vi "Get Base Protocol.vi"(8 "error in (no error)":errorcluster, 11 "UDP in":refnum<class "UDP.lvclass">) -> (0 "error out":errorcluster, 2 "Protocol out":T1, 3 "UDP out":refnum<class "UDP.lvclass">)   [LabVIEW 2019, in "Protocols.lvlib" / "UDP.lvclass"]
uses:
  UDP.lvclass
  Protocol Parent/Types/Base Protocol Type.ctl
  Protocol Parent/Protocol Parent.lvclass
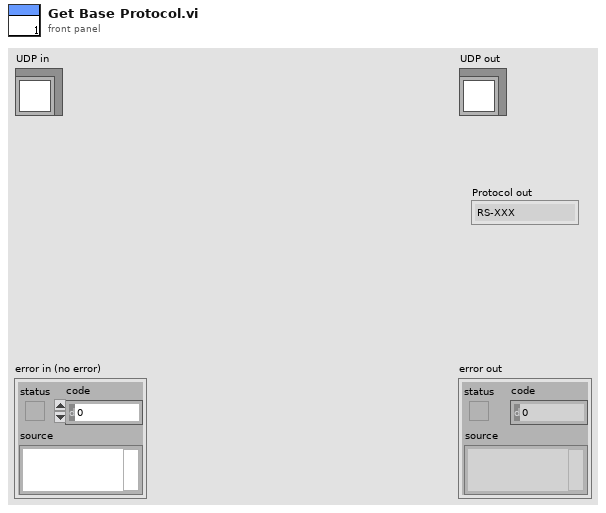
[diagram p1: front panel]
types:
  T1 = typedef "Protocols.lvlib/Protocol Parent.lvclass/Base Protocol Type.ctl" = enum16{"RS-XXX", "VISA", "TCPIP", "UDP"}
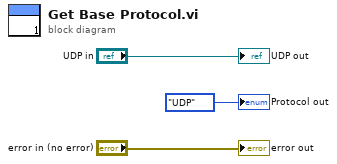
[diagram p0: block diagram]
diagram:
  "error out" <- "error in (no error)"
  "UDP out" <- "UDP in"
  "Protocol out" <- Base_Protocol_Type."UDP" ("Protocol out")
